vi "Read IVI Resource.vi"(8 "error in (no error)":errorcluster, 11 "PXIe5413 in":refnum<class "PXIe5413.lvclass">) -> (0 "error out":errorcluster, 2 "IVI Resource":refnum<k15>, 3 "PXIe5413 out":refnum<class "PXIe5413.lvclass">)   [LabVIEW 2018, in "PXIe5413.lvlib" / "PXIe5413.lvclass"]
uses:
  PXIe5413.lvclass
  PXIe5413.lvclass/PXIe5413.ctl
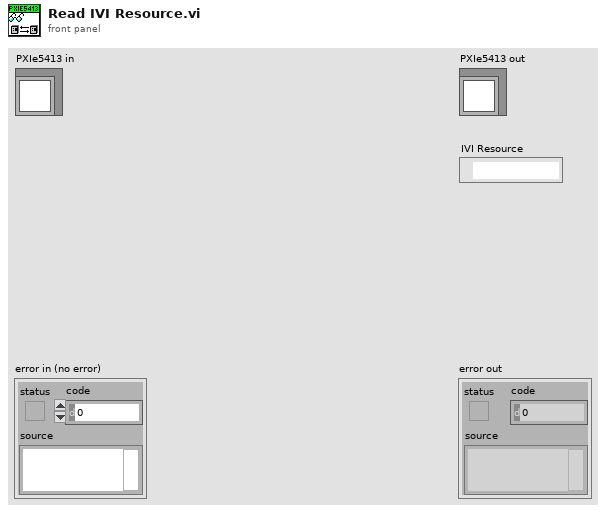
[diagram p1: front panel]
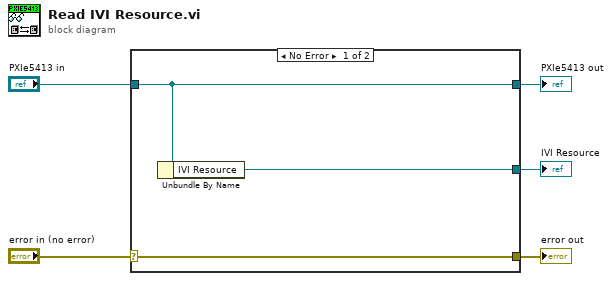
[diagram p0: block diagram]
diagram:
  n1 = case shown="No Error" "error in (no error)" {
    selector: "error in (no error)" -> [w8 w9]
    tunnel: [w8 w9] -> w4
    tunnel: [w7 w10] -> w2
    tunnel: "PXIe5413 in" -> [w7 w10]
    tunnel: [w6 _] -> w1
    frame No Error {
      n2 = Unbundle By Name(w7) -> ("IVI Resource"=w6:refnum<k15>)
    }
    frame Error {
    }
  }
  "error out" <- w4
  "PXIe5413 out" <- w2
  "IVI Resource" <- w1
